vi "S4GUI_001.vi"() -> ()   [LabVIEW 2018] (continued)
      tunnel: "Observer" -> [_ _ _ _ _ _ _ _ _ _ _ _ _ _ _ _ _ _ _ _ _ _ _ _ w3244 _ _ _ _ w5070 w5251 w5440 _ _ w5832 w6021 w6150 w6276 w6403 _ _ _ _ _ _ _ _ _ _ _ _ _ _ _ _ _ _ _ _ _ _ _ _ _ _ _ _ _ _ _ _ _ _ _ _ _ _ _ _ _ _ _ _ _ _ _ _ _ _ _ _ _ _ _ _ _ _ _ _ _ _ _ _ _ _ _ _ _ _ _]
      tunnel: w48 -> [w107 _ _ _ _ _ _ _ _ _ _ _ _ _ _ _ _ _ _ _ _ _ _ _ _ _ _ _ _ _ _ _ _ _ _ _ _ _ _ _ _ _ _ _ _ _ _ _ _ _ _ _ _ _ _ _ _ _ _ _ _ _ _ _ _ _ _ _ _ _ _ _ _ _ _ _ _ _ _ _ _ _ _ _ _ _ _ _ _ _ _ _ _ _ _ _ _ _ _ _ _ _ _ _ _ _ _ _ _ _]
      tunnel: "Tab Acq Type" -> [_ _ _ _ _ _ _ _ _ _ _ _ _ _ _ _ _ _ _ _ _ _ _ _ w3236 _ _ _ _ _ _ _ _ _ _ w6010 _ _ _ _ _ _ _ _ _ _ _ _ _ _ _ _ _ _ _ _ _ _ _ _ _ _ _ _ _ _ _ _ _ _ _ _ _ _ _ _ _ _ _ _ _ _ _ _ _ _ _ _ _ _ _ _ _ _ _ _ _ _ _ _ _ _ _ _ _ _ _ _ _ _]
      event Timeout {
        # "Obtém os valores de status dos\ndispositivos de cada servidor para\napresentar nos indicadores da GUI."
        # "Trata as tarefas individuais de \ncada servidor (ACS1,...,ACS4, \nICS, TCS, SyncBox)"
        # "Determina a sequência de\ntarefas dos servidores\npara uma observação, de \nacordo com o modo de \noperação (disparado com \nos botões START)"
        # "execução dos botões\n no modo sincrono."
        # "execução dos botões\n no modo assincrono."
        # "Instrument States.<device> State\n\n0: nao fez INIT e está parado (mode = IDLE ou WAITING\n                                                    contdition = default)\n1: nao fez INIT e está movendo (mode = IDLE ou WAITING\n                                                    contdition = BUSY)\n\n2: fez INIT e está parado (mode = default)\n                                            condition = READY)\n3: fez INIT e está movendo (mode = default)\n                                            condition = BUSY)"
        n76 = event-data() -> ()  [unwired: 1 in, 2 out]
        n77 = disable-structure shown="Enabled" {
          disable-tunnel: w138 -> [w146 w151]
          disable-tunnel: w137 -> [w145 w149]
          disable-tunnel: [w143 w148] -> w126
          disable-tunnel: [w142 w147] -> w125
          disable-tunnel: w107 -> [_ w150]
          frame Disabled {
            n78 = call "Elapsed Time"() -> ("Time has Elapsed"=w141:bool)  [unwired: 12 in, 7 out]
            n79 = call "Elapsed Time3"() -> ("Time has Elapsed"=w144:bool)  [unwired: 12 in, 7 out]
            n80 = call "Write Status_timeout.vi"("error in (no error)"=w145, "TCS_timeout"=w144, "Status_timeout"=w141, "S4ACS_GUI in"=w146) -> ("error out"=w143:errorcluster, "S4ACS_GUI out"=w142:refnum<class "S4GUI.lvclass">)  [unwired: 6 in]
          }
          frame Enabled {
            n81 = call-dynamic "Write loop counter.vi"("error in (no error)"=w149, "loop counter"=w150, "S4GUI in"=w151) -> ("error out"=w148:errorcluster, "S4GUI out"=w147:refnum<class "S4GUI.lvclass">)  [unwired: 7 in]
          }
        }
        n82 = call-dynamic "HandlePauseAsync.vi"("error in (no error)"=w126, "S4GUI in"=w125) -> ("error out"=w122:errorcluster, "S4GUI out"=w124:refnum<class "S4GUI.lvclass">)  [unwired: 8 in]
        n83 = call-dynamic "HandleStopAsync.vi"("error in (no error)"=w122, "S4GUI in"=w124) -> ("error out"=w121:errorcluster, "S4GUI out"=w123:refnum<class "S4GUI.lvclass">)  [unwired: 8 in]
        n84 = call-dynamic "HandleAbortAsync.vi"("error in (no error)"=w121, "S4GUI in"=w123) -> ("error out"=w115:errorcluster, "S4GUI out"=w116:refnum<class "S4GUI.lvclass">)  [unwired: 8 in]
        n85 = call-dynamic "HandlePauseSync.vi"("error in (no error)"=w115, "S4GUI in"=w116) -> ("error out"=w114:errorcluster, "S4GUI out"=w113:refnum<class "S4GUI.lvclass">)  [unwired: 8 in]
        n86 = call-dynamic "HandleStopSync.vi"("error in (no error)"=w114, "S4GUI in"=w113) -> ("error out"=w118:errorcluster, "S4GUI out"=w120:refnum<class "S4GUI.lvclass">)  [unwired: 8 in]
        n87 = call-dynamic "HandleAbortSync.vi"("error in (no error)"=w118, "S4GUI in"=w120) -> ("error out"=w117:errorcluster, "S4GUI out"=w119:refnum<class "S4GUI.lvclass">)  [unwired: 8 in]
        n88 = call-dynamic "HandleObservation.vi"("error in (no error)"=w117, "S4ACS_GUI in"=w119) -> ("error out"=w131:errorcluster, "S4ACS_GUI out"=w132:refnum<class "S4GUI.lvclass">)  [unwired: 8 in]
        n89 = call-dynamic "HandleServers.vi"("error in (no error)"=w131, "S4ACS_GUI in"=w132) -> ("error out"=w140:errorcluster, "S4ACS_GUI out"=w139:refnum<class "S4GUI.lvclass">)  [unwired: 8 in]
        n90 = call-dynamic "GetStatus.vi"("error in (no error)"=w140, "S4ACS_GUI in"=w139) -> ("error out"=w128:errorcluster, "output cluster"=w133:T9, "Cluster Disable"=w130:T10, "S4ACS_GUI out"=w129:refnum<class "S4GUI.lvclass">)  [unwired: 6 in]
        n91 = call "Elapsed Time2"() -> ("Time has Elapsed"=w112:bool)  [unwired: 12 in, 7 out]
        n92 = call "Read cfg file.vi"("error in (no error)"=w128, "S4ACS_GUI in"=w129) -> ("error out"=w110:errorcluster, "cfg file"=w127:string, "S4ACS_GUI out"=w111:refnum<class "S4GUI.lvclass">)  [unwired: 7 in]
        n93 = case shown="True" w112 {
          selector: w112 -> [_ w180]
          tunnel: w133 -> [_ w183]
          tunnel: w130 -> [_ w182]
          tunnel: w127 -> [_ w181]
          tunnel: w111 -> [w153 w179]
          tunnel: w110 -> [w152 w178]
          tunnel: [w153 w176] -> w109
          tunnel: [w152 w173] -> w108
          frame False {
          }
          frame True {
            # "MODE:\nF -> photometric\nT -> polarimetric"
            n94 = stacked-sequence {
              tunnel: w183 -> [w279 w280 w282 w284 w291 w321 w325 w474 w574 w829 _ _ _ _ _ w1039 w1199 w1332 w1465]
              tunnel: [_ _ _ _ _ _ _ w472 _ _ _ _ _ _ _ _ _ _ _] -> w157
              tunnel: w182 -> [_ _ _ _ _ _ _ _ _ _ w853 w902 w919 w936 w953 _ _ _ _]
              tunnel: w180 -> [_ _ _ _ _ _ w322 _ w569 _ _ _ _ _ _ _ _ _ _]
              tunnel: w181 -> [_ _ _ _ _ _ _ _ _ _ _ _ _ _ _ w1034 _ _ _]
              frame #0 {
                w241 = u32 240 ("Tab Control Pane Dimension:Width")
                w242 = u32 300 ("Tab Control Pane Dimension:Height")
                n95 = Unbundle By Name(w279) -> ("TCS id"=w239:u32, "TCSPD_connection"=→"TCSPD":bool, "TCS extended"=w276:string)
                n96 = Equal?(x=u32 8 ("Tab Control Pane Dimension:Width"), y=w239) -> (x = y?=w238:bool)
                n97 = Match Pattern(string=w276, regular expression="RA=") -> (after substring=w272:string)  [unwired: 1 in, 3 out]
                n98 = local write "TCS mode"(w238) -> ()
                n99 = Match Pattern(string=w272, regular expression="DEC=") -> (before substring=→"RA":string, after substring=w271:string)  [unwired: 1 in, 2 out]
                n100 = Match Pattern(string=w271, regular expression="EQUINOX=") -> (before substring=→"DEC":string, after substring=w270:string)  [unwired: 1 in, 2 out]
                n101 = Match Pattern(string=w270, regular expression="AIRMASS=") -> (after substring=w266:string)  [unwired: 1 in, 3 out]
                n102 = Match Pattern(string=w266, regular expression="TCSHA=") -> (before substring=→"Air Mass":string, after substring=w265:string)  [unwired: 1 in, 2 out]
                n103 = Match Pattern(string=w265, regular expression="TCSDATE=") -> (before substring=→"Hour Angle":string, after substring=w263:string)  [unwired: 1 in, 2 out]
                n104 = Match Pattern(string=w263, regular expression="TELFOCUS=") -> (before substring=→"Date":string, after substring=w259:string)  [unwired: 1 in, 2 out]
                n105 = Match Pattern(string=w259, regular expression="EXTTEMP=") -> (before substring=→"Telescope Focus":string, after substring=w258:string)  [unwired: 1 in, 2 out]
                n106 = Match Pattern(string=w258, regular expression="PRESSURE=") -> (before substring=→"Outside Temp":string, after substring=w257:string)  [unwired: 1 in, 2 out]
                n107 = property on="Tab CH2" class="TabCtl (strict)"("PaneHeight"=w242, "PaneWidth"=w241) -> ()  [unwired: 2 in, 2 out]
                n108 = property on="Tab CH1" class="TabCtl (strict)"("PaneHeight"=w242, "PaneWidth"=w241) -> ()  [unwired: 2 in, 2 out]
                n109 = property on="Tab CH3" class="TabCtl (strict)"("PaneHeight"=w242, "PaneWidth"=w241) -> ()  [unwired: 2 in, 2 out]
                n110 = Match Pattern(string=w257, regular expression="HUMIDITY=") -> (before substring=→"Pressure":string, after substring=w246:string)  [unwired: 1 in, 2 out]
                n111 = property on="Tab CH4" class="TabCtl (strict)"("PaneHeight"=w242, "PaneWidth"=w241) -> ()  [unwired: 2 in, 2 out]
                n112 = Match Pattern(string=w246, regular expression="JD=") -> (before substring=→"Humidity":string, after substring=w247:string)  [unwired: 1 in, 2 out]
                n113 = Match Pattern(string=w247, regular expression="SD=") -> (before substring=→"Julian Date":string, after substring=→"Sideral Time":string)  [unwired: 1 in, 2 out]
              }
              frame #1 {
                n114 = Unbundle By Name(w280) -> ()  [unwired: 1 out]
              }
              frame #2 {
                n115 = Unbundle By Name(w282) -> ("Trigger Mode Status"=→"String":string)
              }
              frame #3 {
                n116 = Unbundle By Name(w284) -> ("Trigger General Status"=→"String 2":string)
              }
              frame #4 {
                n117 = Unbundle By Name(w291) -> ("Instrument Status"=w290:T11, "Instrument States.WPROT State"=w289:i32, "Instrument Pos Names.WPROT posname"=w288:string, "Instrument Pos Names.WPSEL posname"=w287:string, "Instrument Pos Names.CALW posname"=w286:string, "Instrument Pos Names.ASEL posname"=w285:string)
                n118 = stacked-sequence {
                  tunnel: w290 -> [w298 w301 w304 w306 w308 w311 w314 w316 w318]
                  tunnel: w289 -> [w294 _ _ _ _ _ _ _ _]
                  tunnel: w288 -> [_ w299 _ _ _ _ _ _ _]
                  tunnel: w287 -> [_ _ w302 _ _ _ _ _ _]
                  tunnel: w286 -> [_ _ _ _ _ w309 _ _ _]
                  tunnel: w285 -> [_ _ _ _ _ _ w312 _ _]
                  frame #0 {
                    # "Pisca quando BUSY"
                    n119 = Unbundle By Name(w298) -> ("WPROT pos"=w295:dbl)
                    "WaveplatePos 2" <- w295
                    n120 = Equal?(x=w294, y=3) -> (x = y?=w292:bool)
                    n121 = property on="WaveplatePos 2" class="DigNum (strict)"("Blinking"=w292) -> ()  [unwired: 2 in, 2 out]
                    n122 = Number To Fractional String(number=w295, precision (6)=i16 1) -> (F-format string=→"Angle":string)  [unwired: 2 in]
                  }
                  frame #1 {
                    n123 = Unbundle By Name(w301) -> ("WPROT pos"=→"Position WPROT":dbl)
                    "PosName WPROT" <- w299
                  }
                  frame #2 {
                    n124 = Unbundle By Name(w304) -> ("WPSEL pos"=→"Position WPSEL":dbl)
                    "PosName WPSEL" <- w302
                  }
                  frame #3 {
                    n125 = Unbundle By Name(w306) -> ("GMIR pos"=→"Position GMIR":dbl)
                  }
                  frame #4 {
                    n126 = Unbundle By Name(w308) -> ("GFOC pos"=→"Position GFOC":dbl)
                  }
                  frame #5 {
                    n127 = Unbundle By Name(w311) -> ("CALW pos"=→"Position CALW":dbl)
                    "PosName CALW" <- w309
                  }
                  frame #6 {
                    n128 = Unbundle By Name(w314) -> ("ASEL pos"=→"PosName ASEL":dbl)
                    "PosName ASEL" <- w312
                  }
                  frame #7 {
                    n129 = Unbundle By Name(w316) -> ("connection"=→"S4ICSoft":bool)
                  }
                  frame #8 {
                    n130 = Unbundle By Name(w318) -> ("String Status"=→"Status":string)
                  }
                }
              }
              frame #5 {
                n131 = Unbundle By Name(w321) -> ("Sync Box State"=→"Current State":i32, "Trigger_connection"=→"Sync Box" →"LedExtSync":bool)
              }
              frame #6 {
                n132 = Unbundle By Name(w325) -> ("Instrument States"=w324:T12, "Instrument Pos Names"=w323:T13)
                n133 = stacked-sequence {
                  tunnel: w324 -> [w334 w360 w379 w418 w447 w461]
                  tunnel: w323 -> [w330 _ w377 w414 _ _]
                  tunnel: w322 -> [w328 _ w371 w411 _ _]
                  frame #0 {
                    # "WPSEL"
                    n134 = Unbundle By Name(w330) -> ("WPSEL posname"=w326:string)
                    n135 = Unbundle By Name(w334) -> ("WPSEL State"=w333:i32)
                    n136 = local read "WPSEL Status"() -> (w329:bool)
                    n137 = case shown="2" w333 {
                      tunnel: [cluster{u32, u32}[] [{9868950, 9868950}, {9868950, 9868950}] ("Colors [4]") cluster{u32, u32}[] [{9868950, 9868950}, {9868950, 9868950}] ("Colors [4]") cluster{u32, u32}[] [{16318208, 16318208}, {16318208, 16318208}] ("Colors [4]") cluster{u32, u32}[] [{6618880, 2424594}, {6618880, 2424594}] ("Colors [4]") w349] -> w332
                      tunnel: [FALSE ("WPROT Status") FALSE ("WPROT Status") TRUE ("WPROT Status") FALSE ("WPROT Status") w351] -> w331
                      tunnel: w329 -> [_ _ _ _ w350]
                      tunnel: w328 -> [_ _ _ _ w348]
                      tunnel: ["" "" "" w344 ""] -> w327
                      tunnel: w326 -> [_ _ _ w344 _]
                      frame Default {
                      }
                      frame 0 {
                      }
                      frame 1 {
                      }
                      frame 2 {
                      }
                      frame 3 {
                        n138 = case shown="True" w350 {
                          tunnel: [cluster{u32, u32}[] [{7563008, 7563008}, {7563008, 7563008}] ("Colors [4]") cluster{u32, u32}[] [{16318208, 16318208}, {16318208, 16318208}] ("Colors [4]")] -> w349
                          frame False {
                          }
                          frame True {
                          }
                        }
                        n139 = case shown="True" w348 {
                          tunnel: [w352 w354] -> w351
                          tunnel: w350 -> [w352 w353]
                          frame False {
                          }
                          frame True {
                            n140 = Not(x=w353) -> (.not. x?=w354:bool)
                          }
                        }
                      }
                    }
                    "WPSEL Status" <- w331
                    "Waveplate" <- w331
                    n141 = property on="Waveplate" class="Bool (strict)"("Colors [4]"=w332, "BoolText.Text"=w327) -> ()  [unwired: 2 in, 2 out]
                    n142 = property on="WPSEL Status" class="Bool (strict)"("Colors [4]"=w332) -> ()  [unwired: 2 in, 2 out]
                  }
                  frame #1 {
                    # "WPROT"
                    n143 = Unbundle By Name(w360) -> ("WPROT State"=w359:i32)
                    n144 = case shown="2" w359 {
                      tunnel: [cluster{u32, u32}[] [{9868950, 9868950}, {9868950, 9868950}] ("Colors [4]") cluster{u32, u32}[] [{9868950, 9868950}, {9868950, 9868950}] ("Colors [4]") cluster{u32, u32}[] [{16318208, 16318208}, {16318208, 16318208}] ("Colors [4]") cluster{u32, u32}[] [{6618880, 6618880}, {6618880, 6618880}] ("Colors [4]") cluster{u32, u32}[] [{16318208, 16318208}, {16318208, 16318208}] ("Colors [4]")] -> w358
                      tunnel: [FALSE ("WPROT Status") FALSE ("WPROT Status") TRUE ("WPROT Status") FALSE ("WPROT Status") TRUE ("WPROT Status")] -> w357
                      frame Default {
                      }
                      frame 0 {
                      }
                      frame 1 {
                      }
                      frame 2 {
                      }
                      frame 3 {
                      }
                    }
                    "WPROT Status" <- w357
                    n145 = property on="WPROT Status" class="Bool (strict)"("Colors [4]"=w358) -> ()  [unwired: 2 in, 2 out]
                  }
                  frame #2 {
                    # "CALW"
                    n146 = Unbundle By Name(w379) -> ("CALW State"=w378:i32)
                    n147 = Unbundle By Name(w377) -> ("CALW posname"=w376:string)
                    n148 = local read "CALW Status"() -> (w372:bool)
                    n149 = case shown="Default" w378 {
                      tunnel: [cluster{u32, u32}[] [{9868950, 9868950}, {9868950, 9868950}] ("Colors [4]") cluster{u32, u32}[] [{9868950, 9868950}, {9868950, 9868950}] ("Colors [4]") cluster{u32, u32}[] [{16318208, 16318208}, {16318208, 16318208}] ("Colors [4]") cluster{u32, u32}[] [{6618880, 6618880}, {6618880, 6618880}] ("Colors [4]") w400] -> w373
                      tunnel: [FALSE ("WPROT Status") FALSE ("WPROT Status") TRUE ("WPROT Status") FALSE ("WPROT Status") w402] -> w375
                      tunnel: w376 -> [_ _ _ w390 _]
                      tunnel: ["" "" "" w389 ""] -> w374
                      tunnel: w372 -> [_ _ _ _ w401]
                      tunnel: w371 -> [_ _ _ _ w399]
                      frame Default {
                      }
                      frame 0 {
                      }
                      frame 1 {
                      }
                      frame 2 {
                        n150 = case shown="\"SHUTTER\"" w390 {
                          tunnel: ["" "DEPOL" "POL" "OFF" "PIN" "SHT"] -> w389
                          frame Default {
                          }
                          frame "DEPOLARIZER" {
                          }
                          frame "POLARIZER" {
                          }
                          frame "OFF" {
                          }
                          frame "PINHOLE" {
                          }
                          frame "SHUTTER" {
                          }
                        }
                      }
                      frame 3 {
                        n151 = case shown="False" w401 {
                          tunnel: [cluster{u32, u32}[] [{7563008, 7563008}, {7563008, 7563008}] ("Colors [4]") cluster{u32, u32}[] [{16318208, 16318208}, {16318208, 16318208}] ("Colors [4]")] -> w400
                          frame False {
                          }
                          frame True {
                          }
                        }
                        n152 = case shown="True" w399 {
                          tunnel: [w404 w406] -> w402
                          tunnel: w401 -> [w404 w405]
                          frame False {
                          }
                          frame True {
                            n153 = Not(x=w405) -> (.not. x?=w406:bool)
                          }
                        }
                      }
                    }
                    "CALW Status" <- w375
                    "PCS" <- w375
                    n154 = property on="CALW Status" class="Bool (strict)"("Colors [4]"=w373) -> ()  [unwired: 2 in, 2 out]
                    n155 = property on="PCS" class="Bool (strict)"("Colors [4]"=w373, "BoolText.Text"=w374) -> ()  [unwired: 2 in, 2 out]
                  }
                  frame #3 {
                    # "ASEL"
                    n156 = Unbundle By Name(w418) -> ("ASEL State"=w417:i32)
                    n157 = Unbundle By Name(w414) -> ("ASEL posname"=w410:string)
                    n158 = local read "ASEL Status"() -> (w412:bool)
                    n159 = case shown="Default" w410 {
                      selector: w410 -> [w419 _ _]
                      tunnel: [w419 "OFF" ("y") "ON" ("y")] -> w409
                      frame Default {
                      }
                      frame "OFF" {
                      }
                      frame "ON" {
                      }
                    }
                    n160 = case shown="2" w417 {
                      tunnel: [cluster{u32, u32}[] [{9868950, 9868950}, {9868950, 9868950}] ("Colors [4]") cluster{u32, u32}[] [{9868950, 9868950}, {9868950, 9868950}] ("Colors [4]") cluster{u32, u32}[] [{16318208, 16318208}, {16318208, 16318208}] ("Colors [4]") cluster{u32, u32}[] [{6618880, 6618880}, {6618880, 6618880}] ("Colors [4]") w438] -> w415
                      tunnel: [FALSE ("WPROT Status") FALSE ("WPROT Status") TRUE FALSE ("WPROT Status") w437] -> w416
                      tunnel: w409 -> [_ _ _ w432 _]
                      tunnel: ["" ("y") "" ("y") "" ("y") w432 "" ("y")] -> w413
                      tunnel: w412 -> [_ _ _ _ w435]
                      tunnel: w411 -> [_ _ _ _ w434]
                      frame Default {
                      }
                      frame 0 {
                      }
                      frame 1 {
                      }
                      frame 2 {
                      }
                      frame 3 {
                        n161 = case shown="True" w435 {
                          tunnel: [cluster{u32, u32}[] [{7563008, 7563008}, {7563008, 7563008}] ("Colors [4]") cluster{u32, u32}[] [{16318208, 16318208}, {16318208, 16318208}] ("Colors [4]")] -> w438
                          frame False {
                          }
                          frame True {
                          }
                        }
                        n162 = case shown="True" w434 {
                          tunnel: [w439 w441] -> w437
                          tunnel: w435 -> [w439 w440]
                          frame False {
                          }
                          frame True {
                            n163 = Not(x=w440) -> (.not. x?=w441:bool)
                          }
                        }
                      }
                    }
                    "ASEL Status" <- w416
                    "Analyzer" <- w416
                    n164 = property on="Analyzer" class="Bool (strict)"("Colors [4]"=w415, "BoolText.Text"=w413) -> ()  [unwired: 2 in, 2 out]
                    n165 = property on="ASEL Status" class="Bool (strict)"("Colors [4]"=w415) -> ()  [unwired: 2 in, 2 out]
                  }
                  frame #4 {
                    # "GMIR"
                    n166 = Unbundle By Name(w447) -> ("GMIR State"=w446:i32)
                    n167 = case shown="2" w446 {
                      tunnel: [cluster{u32, u32}[] [{9868950, 9868950}, {9868950, 9868950}] ("Colors [4]") cluster{u32, u32}[] [{9868950, 9868950}, {9868950, 9868950}] ("Colors [4]") cluster{u32, u32}[] [{16318208, 16318208}, {16318208, 16318208}] ("Colors [4]") cluster{u32, u32}[] [{6618880, 6618880}, {6618880, 6618880}] ("Colors [4]") cluster{u32, u32}[] [{16318208, 16318208}, {16318208, 16318208}] ("Colors [4]")] -> w445
                      tunnel: [FALSE ("WPROT Status") FALSE ("WPROT Status") TRUE ("WPROT Status") FALSE ("WPROT Status") TRUE ("WPROT Status")] -> w444
                      frame Default {
                      }
                      frame 0 {
                      }
                      frame 1 {
                      }
                      frame 2 {
                      }
                      frame 3 {
                      }
                    }
                    "GMIR Status" <- w444
                    n168 = property on="GMIR Status" class="Bool (strict)"("Colors [4]"=w445) -> ()  [unwired: 2 in, 2 out]
                  }
                  frame #5 {
                    # "GFOC"
                    n169 = Unbundle By Name(w461) -> ("GFOC State"=w460:i32)
                    n170 = case shown="0" w460 {
                      tunnel: [cluster{u32, u32}[] [{9868950, 9868950}, {9868950, 9868950}] ("Colors [4]") cluster{u32, u32}[] [{9868950, 9868950}, {9868950, 9868950}] ("Colors [4]") cluster{u32, u32}[] [{16318208, 16318208}, {16318208, 16318208}] ("Colors [4]") cluster{u32, u32}[] [{6618880, 6618880}, {6618880, 6618880}] ("Colors [4]") cluster{u32, u32}[] [{16318208, 16318208}, {16318208, 16318208}] ("Colors [4]")] -> w459
                      tunnel: [FALSE ("WPROT Status") FALSE ("WPROT Status") TRUE ("WPROT Status") FALSE ("WPROT Status") TRUE ("WPROT Status")] -> w458
                      frame Default {
                      }
                      frame 0 {
                      }
                      frame 1 {
                      }
                      frame 2 {
                      }
                      frame 3 {
                      }
                    }
                    "GFOC Status" <- w458
                    n171 = property on="GFOC Status" class="Bool (strict)"("Colors [4]"=w459) -> ()  [unwired: 2 in, 2 out]
                  }
                }
              }
              frame #7 {
                n172 = Unbundle By Name(w474) -> ("Instrument Pos Names"=w473:T13)
                n173 = stacked-sequence {
                  tunnel: w473 -> [w476 w493 w518 w544]
                  tunnel: [_ _ _ w545] -> w472
                  frame #0 {
                    n174 = Unbundle By Name(w476) -> ("WPSEL posname"=w475:string)
                    n175 = case shown="\"L/2\", \"L/4\", \"OFF\"" w475 {
                      selector: w475 -> [_ w477]
                      frame "False", Default {
                      }
                      frame "L/2", "L/4", "OFF" {
                        n176 = First Call?() -> (First Call?: T/F=w478:bool)
                        n177 = case shown="True" w478 {
                          tunnel: w477 -> [_ w479]
                          frame False {
                          }
                          frame True {
                            n178 = case shown="\"L/2\"" w479 {
                              frame "False", Default {
                              }
                              frame "L/2" {
                                w480 = u16 1 items=["OFF", "Lambda/2", "Lambda/4"] ("Lambda Selector")
                                n179 = property on="Lambda Selector" class="Ring (strict)"(error in=errorcluster {"status"=FALSE, "code"=0, "source"=""} ("error in (no error)"), "Value"=w480) -> (error out=w482:errorcluster)  [unwired: 1 in, 1 out]
                                n180 = property on="Lambda Selector" class="Ring (strict)"(error in=w482, "RingText.Text"="Lambda/2" ("Boolean Text.Text")) -> ()  [unwired: 1 in, 2 out]
                              }
                              frame "L/4" {
                                w484 = u16 2 items=["OFF", "Lambda/2", "Lambda/4"] ("Lambda Selector")
                                n181 = property on="Lambda Selector" class="Ring (strict)"(error in=errorcluster {"status"=FALSE, "code"=0, "source"=""} ("error in (no error)"), "Value"=w484) -> (error out=w486:errorcluster)  [unwired: 1 in, 1 out]
                                n182 = property on="Lambda Selector" class="Ring (strict)"(error in=w486, "RingText.Text"="Lambda/4" ("Boolean Text.Text")) -> ()  [unwired: 1 in, 2 out]
                              }
                              frame "OFF" {
                                w488 = u16 0 items=["OFF", "Lambda/2", "Lambda/4"] ("Lambda Selector")
                                n183 = property on="Lambda Selector" class="Ring (strict)"(error in=errorcluster {"status"=FALSE, "code"=0, "source"=""} ("error in (no error)"), "Value"=w488) -> (error out=w490:errorcluster)  [unwired: 1 in, 1 out]
                                n184 = property on="Lambda Selector" class="Ring (strict)"(error in=w490, "RingText.Text"="OFF" ("Boolean Text.Text")) -> ()  [unwired: 1 in, 2 out]
                              }
                            }
                          }
                        }
                      }
                    }
                  }
                  frame #1 {
                    n185 = Unbundle By Name(w493) -> ("CALW posname"=w492:string)
                    n186 = case shown="\"DEPOLARIZER\", \"OFF\", \"PINHOLE\", \"POLARIZER\", \"SHUTTER\"" w492 {
                      selector: w492 -> [_ w494]
                      frame "False", Default {
                      }
                      frame "DEPOLARIZER", "OFF", "PINHOLE", "POLARIZER", "SHUTTER" {
                        n187 = First Call?() -> (First Call?: T/F=w495:bool)
                        n188 = case shown="True" w495 {
                          tunnel: w494 -> [_ w496]
                          frame False {
                          }
                          frame True {
                            n189 = case shown="\"OFF\"" w496 {
                              frame "False", Default {
                              }
                              frame "POLARIZER" {
                                w497 = u16 1 items=["OFF", "POLARIZER", "PINHOLE", "SHUTTER", "DEPOLARIZER"] ("Calibrator Selector")
                                n190 = property on="Calibrator Selector" class="Ring (strict)"(error in=errorcluster {"status"=FALSE, "code"=0, "source"=""} ("error in (no error)"), "Value"=w497) -> (error out=w499:errorcluster)  [unwired: 1 in, 1 out]
                                n191 = property on="Calibrator Selector" class="Ring (strict)"(error in=w499, "RingText.Text"="POLARIZER" ("Boolean Text.Text")) -> ()  [unwired: 1 in, 2 out]
                              }
                              frame "DEPOLARIZER" {
                                w501 = u16 4 items=["OFF", "POLARIZER", "PINHOLE", "SHUTTER", "DEPOLARIZER"] ("Calibrator Selector")
                                n192 = property on="Calibrator Selector" class="Ring (strict)"(error in=errorcluster {"status"=FALSE, "code"=0, "source"=""} ("error in (no error)"), "Value"=w501) -> (error out=w503:errorcluster)  [unwired: 1 in, 1 out]
                                n193 = property on="Calibrator Selector" class="Ring (strict)"(error in=w503, "RingText.Text"="DEPOLARIZER" ("Boolean Text.Text")) -> ()  [unwired: 1 in, 2 out]
                              }
                              frame "PINHOLE" {
                                w505 = u16 2 items=["OFF", "POLARIZER", "PINHOLE", "SHUTTER", "DEPOLARIZER"] ("Calibrator Selector")
                                n194 = property on="Calibrator Selector" class="Ring (strict)"(error in=errorcluster {"status"=FALSE, "code"=0, "source"=""} ("error in (no error)"), "Value"=w505) -> (error out=w507:errorcluster)  [unwired: 1 in, 1 out]
                                n195 = property on="Calibrator Selector" class="Ring (strict)"(error in=w507, "RingText.Text"="PINHOLE" ("Boolean Text.Text")) -> ()  [unwired: 1 in, 2 out]
                              }
                              frame "SHUTTER" {
                                w509 = u16 3 items=["OFF", "POLARIZER", "PINHOLE", "SHUTTER", "DEPOLARIZER"] ("Calibrator Selector")
                                n196 = property on="Calibrator Selector" class="Ring (strict)"(error in=errorcluster {"status"=FALSE, "code"=0, "source"=""} ("error in (no error)"), "Value"=w509) -> (error out=w511:errorcluster)  [unwired: 1 in, 1 out]
                                n197 = property on="Calibrator Selector" class="Ring (strict)"(error in=w511, "RingText.Text"="SHUTTER" ("Boolean Text.Text")) -> ()  [unwired: 1 in, 2 out]
                              }
                              frame "OFF" {
                                w513 = u16 0 items=["OFF", "POLARIZER", "PINHOLE", "SHUTTER", "DEPOLARIZER"] ("Calibrator Selector")
                                n198 = property on="Calibrator Selector" class="Ring (strict)"(error in=errorcluster {"status"=FALSE, "code"=0, "source"=""} ("error in (no error)"), "Value"=w513) -> (error out=w515:errorcluster)  [unwired: 1 in, 1 out]
                                n199 = property on="Calibrator Selector" class="Ring (strict)"(error in=w515, "RingText.Text"="OFF" ("Boolean Text.Text")) -> ()  [unwired: 1 in, 2 out]
                              }
                            }
                          }
                        }
                      }
                    }
                  }
                  frame #2 {
                    n200 = Unbundle By Name(w518) -> ("WPROT posname"=w517:string)
                    "Name" <- w517
                    n201 = stacked-sequence {
                      tunnel: w517 -> [_ w520]
                      frame #0 {
                        w519 = FALSE
                        "ledP0" <- w519
                        "ledP1" <- w519
                        "ledP2" <- w519
                        "ledP3" <- w519
                        "ledP4" <- w519
                        "ledP5" <- w519
                        "ledP6" <- w519
                        "ledP7" <- w519
                        "ledP8" <- w519
                        "ledP9" <- w519
                        "ledP10" <- w519
                        "ledP11" <- w519
                        "ledP12" <- w519
                        "ledP13" <- w519
                        "ledP14" <- w519
                        "ledP15" <- w519
                      }
                      frame #1 {
                        n202 = case shown="\"WP15\"" w520 {
                          frame Default {
                          }
                          frame "WP1" {
                            n203 = local write "ledP0"(TRUE ("ledP0")) -> ()
                          }
                          frame "WP2" {
                            n204 = local write "ledP1"(TRUE ("ledP0")) -> ()
                          }
                          frame "WP3" {
                            n205 = local write "ledP2"(TRUE ("ledP0")) -> ()
                          }
                          frame "WP4" {
                            n206 = local write "ledP3"(TRUE ("ledP0")) -> ()
                          }
                          frame "WP5" {
                            n207 = local write "ledP4"(TRUE ("ledP0")) -> ()
                          }
                          frame "WP6" {
                            n208 = local write "ledP5"(TRUE ("ledP0")) -> ()
                          }
                          frame "WP7" {
                            n209 = local write "ledP6"(TRUE ("ledP0")) -> ()
                          }
                          frame "WP8" {
                            n210 = local write "ledP7"(TRUE ("ledP0")) -> ()
                          }
                          frame "WP9" {
                            n211 = local write "ledP8"(TRUE ("ledP0")) -> ()
                          }
                          frame "WP10" {
                            n212 = local write "ledP9"(TRUE ("ledP0")) -> ()
                          }
                          frame "WP11" {
                            n213 = local write "ledP10"(TRUE ("ledP0")) -> ()
                          }
                          frame "WP12" {
                            n214 = local write "ledP11"(TRUE ("ledP0")) -> ()
                          }
                          frame "WP13" {
                            n215 = local write "ledP12"(TRUE ("ledP0")) -> ()
                          }
                          frame "WP14" {
                            n216 = local write "ledP13"(TRUE ("ledP0")) -> ()
                          }
                          frame "WP15" {
                            n217 = local write "ledP14"(TRUE ("ledP0")) -> ()
                          }
                          frame "WP16" {
                            n218 = local write "ledP15"(TRUE ("ledP0")) -> ()
                          }
                        }
                      }
                    }
                  }
                  frame #3 {
                    w548 = "OFF" ("Boolean Text.Text")
                    # "Polarimetria:   ASEL = ON  &   (WPSEL =L/2 or L/4)\n\nFotometria:    ASEL=OFF & WPSEL = OFF & CALW = OFF"
                    n219 = Unbundle By Name(w544) -> ("ASEL posname"=w539:string, "WPSEL posname"=w541:string, "ASEL posname"=w540:string)
                    n220 = Unbundle By Name(w544) -> ("WPSEL posname"=w551:string, "CALW posname"=w552:string, "ASEL posname"=w546:string)
                    n221 = Equal?(x=w539, y="ON" ("Boolean Text.Text")) -> (x = y?=w542:bool)
                    n222 = case shown="True" w542 {
                      tunnel: w541 -> [w561 w566]
                      tunnel: w540 -> [w560 _]
                      tunnel: w539 -> [w557 _]
                      tunnel: [FALSE ("Polarimetric Mode") w563] -> w538
                      tunnel: [w553 FALSE ("Photometric Mode")] -> w537
                      frame False {
                        w556 = "OFF" ("Boolean Text.Text")
                        n223 = Equal?(x=w557, y=w556) -> (x = y?=w555:bool)
                        n224 = Equal?(x=w560, y=w556) -> (x = y?=w558:bool)
                        n225 = Equal?(x=w561, y=w556) -> (x = y?=w559:bool)
                        n226 = Compound Arithmetic op=AND(w555, w559, w558) -> (w553:bool)
                      }
                      frame True {
                        n227 = Equal?(x="L/2" ("Boolean Text.Text"), y=w566) -> (x = y?=w567:bool)
                        n228 = Equal?(x="L/4" ("Boolean Text.Text"), y=w566) -> (x = y?=w564:bool)
                        n229 = Or(x=w567, y=w564) -> (x .or. y?=w563:bool)
                      }
                    }
                    "Polarimetric Mode" <- w538
                    "Photometric Mode" <- w537
                    n230 = Equal?(x=w548, y=w551) -> (x = y?=w549:bool)
                    n231 = Equal?(x=w548, y=w552) -> (x = y?=w550:bool)
                    n232 = Equal?(x=w548, y=w546) -> (x = y?=w547:bool)
                    n233 = Compound Arithmetic op=AND(w549, w550, w547) -> (invert w545:bool)
                  }
                }
              }
              frame #8 {
                n234 = Unbundle By Name(w574) -> ("ChannelA_Status"=w573:T14, "ChannelB_Status"=w572:T14, "ChannelC_Status"=w570:T14, "ChannelD_Status"=w571:T14)
                n235 = stacked-sequence {
                  tunnel: w573 -> [w630 w686 w739 w815 _ _ _]
                  tunnel: w572 -> [w629 w684 w738 _ w818 _ _]
                  tunnel: w571 -> [w627 w681 w736 _ _ _ w826]
                  tunnel: w570 -> [w628 w682 w737 _ _ w822 _]
                  tunnel: w569 -> [_ _ w728 _ _ _ _]
                  frame #0 {
                    n236 = Unbundle By Name(w627) -> ("connection"=w603:bool, "FT"=w576:bool, "Current exp"=→"Exposure Time ch4":dbl, "Cooler ON/OFF"=w617:i16, "Currently temperature"=w614:i16, "Temperature Status"=w611:string, "target  temp"=w599:i16)
                    n237 = Unbundle By Name(w629) -> ("connection"=w605:bool, "FT"=w580:bool, "Current exp"=→"Exposure Time ch2":dbl, "Cooler ON/OFF"=w619:i16, "Currently temperature"=w616:i16, "Temperature Status"=w613:string, "target  temp"=w601:i16)
                    n238 = Unbundle By Name(w630) -> ("connection"=w606:bool, "FT"=w581:bool, "Current exp"=→"Exposure Time ch1":dbl, "Cooler ON/OFF"=w622:i16, "Currently temperature"=w620:i16, "Temperature Status"=w621:string, "target  temp"=w602:i16)
                    n239 = Unbundle By Name(w628) -> ("connection"=w604:bool, "FT"=w578:bool, "Current exp"=→"Exposure Time ch3":dbl, "Cooler ON/OFF"=w618:i16, "Currently temperature"=w615:i16, "Temperature Status"=w612:string, "target  temp"=w600:i16)
                    n240 = Not Equal To 0?(x=w617) -> (x != 0?=w608:bool)
                    n241 = First Call?() -> (First Call?: T/F=w598:bool)
                    n242 = First Call?() -> (First Call?: T/F=w596:bool)
                    n243 = First Call?() -> (First Call?: T/F=w595:bool)
                    n244 = Not Equal To 0?(x=w618) -> (x != 0?=w607:bool)
                    n245 = First Call?() -> (First Call?: T/F=w597:bool)
                    n246 = case shown="True" w596 {
                      tunnel: w600 -> [_ w632]
                      frame False {
                      }
                      frame True {
                        n247 = property on="Target Temp 3" class="DigNum (strict)"("Value"=w632) -> ()  [unwired: 2 in, 2 out]
                      }
                    }
                    n248 = case shown="True" w598 {
                      tunnel: w602 -> [_ w634]
                      frame False {
                      }
                      frame True {
                        n249 = property on="Target Temp 1" class="DigNum (strict)"("Value"=w634) -> ()  [unwired: 2 in, 2 out]
                      }
                    }
                    n250 = case shown="True" w595 {
                      tunnel: w599 -> [_ w631]
                      frame False {
                      }
                      frame True {
                        n251 = property on="Target Temp 4" class="DigNum (strict)"("Value"=w631) -> ()  [unwired: 2 in, 2 out]
                      }
                    }
                    n252 = case shown="True" w597 {
                      tunnel: w601 -> [_ w633]
                      frame False {
                      }
                      frame True {
                        n253 = property on="Target Temp 2" class="DigNum (strict)"("Value"=w633) -> ()  [unwired: 2 in, 2 out]
                      }
                    }
                    n254 = Not Equal To 0?(x=w622) -> (x != 0?=w609:bool)
                    n255 = Not Equal To 0?(x=w619) -> (x != 0?=w610:bool)
                    n256 = case shown="True" w606 {
                      tunnel: w621 -> [_ w664]
                      tunnel: w620 -> [_ w665]
                      tunnel: w609 -> [_ w666]
                      tunnel: [FALSE w666] -> w594
                      tunnel: [i16 0 ("Currently temperature") w665] -> w593
                      tunnel: ["" ("Temperature Status") w664] -> w592
                      tunnel: [FALSE w663] -> w582
                      tunnel: w581 -> [_ w663]
                      frame False {
                      }
                      frame True {
                      }
                    }
                    "Cooler status 1" <- w594
                    "Curr Temp 1" <- w593
                    "Temp Status 1" <- w592
                    "Panel Temp" <- w593
                    "Panel cooler 1" <- w594
                    "FT1" <- w582
                    n257 = case shown="True" w605 {
                      tunnel: w616 -> [_ w657]
                      tunnel: w613 -> [_ w656]
                      tunnel: w610 -> [_ w658]
                      tunnel: [FALSE w658] -> w591
                      tunnel: [i16 0 ("Currently temperature") w657] -> w590
                      tunnel: ["" ("Temperature Status") w656] -> w589
                      tunnel: w580 -> [_ w655]
                      tunnel: [FALSE ("FT") w655] -> w579
                      frame False {
                      }
                      frame True {
                      }
                    }
                    "Panel Temp 2" <- w590
                    "Curr Temp 2" <- w590
                    "Cooler status 2" <- w591
                    "Panel cooler 2" <- w591
                    "Temp Status 2" <- w589
                    "FT2" <- w579
                    n258 = case shown="True" w603 {
                      tunnel: w614 -> [_ w641]
                      tunnel: w611 -> [_ w640]
                      tunnel: w608 -> [_ w642]
                      tunnel: [FALSE w642] -> w585
                      tunnel: [i16 0 ("Currently temperature") w641] -> w584
                      tunnel: ["" ("Temperature Status") w640] -> w583
                      tunnel: w576 -> [_ w639]
                      tunnel: [FALSE ("FT") w639] -> w575
                      frame False {
                      }
                      frame True {
                      }
                    }
                    "Cooler status 4" <- w585
                    "Panel Temp 4" <- w584
                    "Curr Temp 4" <- w584
                    "Temp Status 4" <- w583
                    "Panel cooler 4" <- w585
                    "FT4" <- w575
                    n259 = case shown="True" w604 {
                      tunnel: w615 -> [_ w649]
                      tunnel: w612 -> [_ w648]
                      tunnel: w607 -> [_ w650]
                      tunnel: [FALSE w650] -> w588
                      tunnel: [i16 0 ("Currently temperature") w649] -> w587
                      tunnel: ["" ("Temperature Status") w648] -> w586
                      tunnel: w578 -> [_ w647]
                      tunnel: [FALSE ("FT") w647] -> w577
                      frame False {
                      }
                      frame True {
                      }
                    }
                    "Cooler status 3" <- w588
                    "Panel Temp 3" <- w587
                    "Curr Temp 3" <- w587
                    "Temp Status 3" <- w586
                    "Panel cooler 3" <- w588
                    "FT3" <- w577
                  }
                  frame #1 {
                    n260 = Unbundle By Name(w681) -> ("LastFileImage"=→"Last Image ch4":string, "Temperature Status"=w669:string)
                    n261 = Unbundle By Name(w682) -> ("LastFileImage"=→"Last Image ch3":string, "Temperature Status"=w670:string)
                    n262 = Unbundle By Name(w684) -> ("LastFileImage"=→"Last Image ch2":string, "Temperature Status"=w673:string)
                    n263 = Unbundle By Name(w686) -> ("LastFileImage"=→"Last Image ch1":string, "Temperature Status"=w678:string)
                    n264 = case shown="\"TEMPERATURE_NOT_REACHED\"" w678 {
                      tunnel: [cluster{u32, u32}[] [{6124107, 6124107}, {6124107, 6124107}] ("Colors [4]") cluster{u32, u32}[] [{6618880, 6618880}, {6618880, 6618880}] ("Colors [4]") cluster{u32, u32}[] [{16318208, 16318208}, {16318208, 16318208}] ("Colors [4]") cluster{u32, u32}[] [{8554752, 8554752}, {8554752, 8554752}] ("Colors [4]")] -> w677
                      tunnel: [FALSE FALSE FALSE TRUE] -> w676
                      frame Default {
                      }
                      frame "TEMPERATURE_STABILIZED" {
                      }
                      frame "TEMPERATURE_NOT_STABILIZED" {
                      }
                      frame "TEMPERATURE_NOT_REACHED" {
                      }
                    }
                    n265 = case shown="\"TEMPERATURE_NOT_REACHED\"" w673 {
                      tunnel: [cluster{u32, u32}[] [{6124107, 6124107}, {6124107, 6124107}] ("Colors [4]") cluster{u32, u32}[] [{6618880, 6618880}, {6618880, 6618880}] ("Colors [4]") cluster{u32, u32}[] [{16318208, 16318208}, {16318208, 16318208}] ("Colors [4]") cluster{u32, u32}[] [{8554752, 8554752}, {8554752, 8554752}] ("Colors [4]")] -> w675
                      tunnel: [FALSE FALSE FALSE TRUE] -> w674
                      frame Default {
                      }
                      frame "TEMPERATURE_STABILIZED" {
                      }
                      frame "TEMPERATURE_NOT_STABILIZED" {
                      }
                      frame "TEMPERATURE_NOT_REACHED" {
                      }
                    }
                    n266 = case shown="\"TEMPERATURE_NOT_REACHED\"" w670 {
                      tunnel: [cluster{u32, u32}[] [{6124107, 6124107}, {6124107, 6124107}] ("Colors [4]") cluster{u32, u32}[] [{6618880, 6618880}, {6618880, 6618880}] ("Colors [4]") cluster{u32, u32}[] [{16318208, 16318208}, {16318208, 16318208}] ("Colors [4]") cluster{u32, u32}[] [{8554752, 8554752}, {8554752, 8554752}] ("Colors [4]")] -> w672
                      tunnel: [FALSE FALSE FALSE TRUE] -> w671
                      frame Default {
                      }
                      frame "TEMPERATURE_STABILIZED" {
                      }
                      frame "TEMPERATURE_NOT_STABILIZED" {
                      }
                      frame "TEMPERATURE_NOT_REACHED" {
                      }
                    }
                    n267 = case shown="\"TEMPERATURE_NOT_REACHED\"" w669 {
                      tunnel: [cluster{u32, u32}[] [{6124107, 6124107}, {6124107, 6124107}] ("Colors [4]") cluster{u32, u32}[] [{6618880, 6618880}, {6618880, 6618880}] ("Colors [4]") cluster{u32, u32}[] [{16318208, 16318208}, {16318208, 16318208}] ("Colors [4]") cluster{u32, u32}[] [{8554752, 8554752}, {8554752, 8554752}] ("Colors [4]")] -> w668
                      tunnel: [FALSE FALSE FALSE TRUE] -> w667
                      frame Default {
                      }
                      frame "TEMPERATURE_STABILIZED" {
                      }
                      frame "TEMPERATURE_NOT_STABILIZED" {
                      }
                      frame "TEMPERATURE_NOT_REACHED" {
                      }
                    }
                    n268 = property on="Cooler status 1" class="Bool (strict)"("Colors [4]"=w677, "Blinking"=w676) -> ()  [unwired: 2 in, 2 out]
                    n269 = property on="Panel cooler 1" class="Bool (strict)"("Colors [4]"=w677, "Blinking"=w676) -> ()  [unwired: 2 in, 2 out]
                    n270 = property on="Cooler status 4" class="Bool (strict)"("Colors [4]"=w668, "Blinking"=w667) -> ()  [unwired: 2 in, 2 out]
                    n271 = property on="Cooler status 3" class="Bool (strict)"("Colors [4]"=w672, "Blinking"=w671) -> ()  [unwired: 2 in, 2 out]
                    n272 = property on="Panel cooler 4" class="Bool (strict)"("Colors [4]"=w668, "Blinking"=w667) -> ()  [unwired: 2 in, 2 out]
                    n273 = property on="Cooler status 2" class="Bool (strict)"("Colors [4]"=w675, "Blinking"=w674) -> ()  [unwired: 2 in, 2 out]
                    n274 = property on="Panel cooler 3" class="Bool (strict)"("Colors [4]"=w672, "Blinking"=w671) -> ()  [unwired: 2 in, 2 out]
                    n275 = property on="Panel cooler 2" class="Bool (strict)"("Colors [4]"=w675, "Blinking"=w674) -> ()  [unwired: 2 in, 2 out]
                  }
                  frame #2 {
                    n276 = Unbundle By Name(w738) -> ("CamStatus"=w731:string, "connection"=w724:bool)
                    n277 = Unbundle By Name(w737) -> ("CamStatus"=w733:string, "connection"=w720:bool)
                    n278 = Unbundle By Name(w736) -> ("CamStatus"=w734:string, "connection"=w719:bool)
                    n279 = Unbundle By Name(w739) -> ("CamStatus"=w729:string, "connection"=w726:bool)
                    n280 = case shown="True" w719 {
                      tunnel: [u32 16739417 w745] -> w735
                      tunnel: w734 -> [_ w742]
                      tunnel: w728 -> [_ w743]
                      tunnel: ["" ("CamStatus") w742] -> w721
                      frame False {
                      }
                      frame True {
                        n281 = property on="Acq status string ch4" class="Str"() -> ("Text.BGColor"=w744:u32)  [unwired: 2 in, 2 out]
                        n282 = case shown="Default" w742 {
                          tunnel: [w748 u32 13882323 u32 13882323] -> w745
                          tunnel: w743 -> [w747 _ _]
                          tunnel: w744 -> [w746 _ _]
                          frame Default {
                            n283 = case shown="True" w747 {
                              tunnel: [w749 w753] -> w748
                              tunnel: w746 -> [w749 w750]
                              frame False {
                              }
                              frame True {
                                n284 = Equal?(x=w750, y=u32 16776002) -> (x = y?=w752:bool)
                                n285 = case shown="True" w752 {
                                tunnel: [u32 16776002 u32 9346816] -> w753
                                frame False {
                                }
                                frame True {
                                }
                                }
                              }
                            }
                          }
                          frame "IDLE" {
                          }
                          frame "" {
                            # "sem resposta do ACS"
                          }
